vi "GetURLBody.vi"(9 "Delay (1000)":u32=1000, 10 "Retries (5)":i32=5, 11 "URL":string) -> (0 "error out":errorcluster, 1 "Retries":i32, 2 "Success?":bool, 3 "body":string)   [LabVIEW 2022 SP3]
uses:
  <vilib>/httpClient/LabVIEWHTTPClient.lvlib
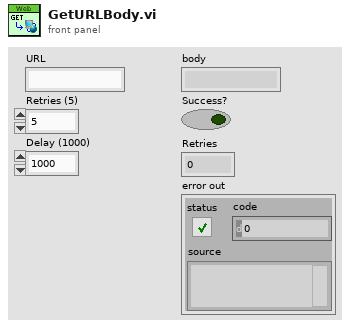
[diagram p1: front panel]
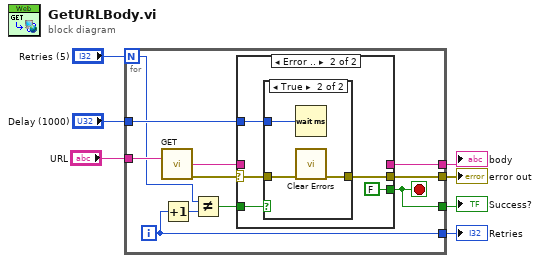
[diagram p0: block diagram]
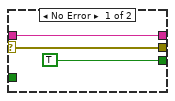
[diagram p2: hidden frame]
diagram:
  n1 = for {
    N: "Retries (5)" -> [w8]
    tunnel: [w17] -> w7
    tunnel: "Delay (1000)" -> [w16]
    tunnel: [w15] -> w6
    tunnel: "URL" -> [w13]
    tunnel: [w12] -> w4
    tunnel: [w11] -> w5
    i -> [w11]
    stop <- w12 stop-if-true
    n2 = call <vilib>:"GET.vi"("url"=w13) -> ("body"=w14:string, "error out"=w18:errorcluster)  [unwired: 11 in, 2 out]
    n3 = Increment(x=w11) -> (x+1=w10:i32)
    n4 = Not Equal?(x=w8, y=w10) -> (x != y?=w9:bool)
    n5 = case shown="Error .." w18 {
      selector: w18 -> [w20 w24]
      tunnel: [TRUE FALSE] -> w12
      tunnel: [w20 w23] -> w17
      tunnel: w16 -> [_ w26]
      tunnel: [w19 _] -> w15
      tunnel: w14 -> [w19 _]
      tunnel: w9 -> [_ w22]
      frame No Error {
      }
      frame Error {
        n6 = case shown="True" w22 {
          tunnel: w26 -> [_ w30]
          tunnel: w24 -> [w27 w29]
          tunnel: [w27 w28] -> w23
          frame False {
          }
          frame True {
            n7 = Wait (ms)(milliseconds to wait=w30) -> ()  [unwired: 1 out]
            n8 = call <vilib>:"Clear Errors.vi"("error in (no error)"=w29) -> ("error out"=w28:errorcluster)  [unwired: 5 in, 1 out]
          }
        }
      }
    }
  }
  "error out" <- w7
  "body" <- w6
  "Retries" <- w5
  "Success?" <- w4
